vi "circle_measurements.vi"(0 "Radius":dbl) -> (1 "Area":dbl, 2 "Circumference":dbl, 3 "Diameter":dbl)   [LabVIEW 2010]
doc: "Given the radius r, this vi calculates the diameter, circumference, and area of the circle"
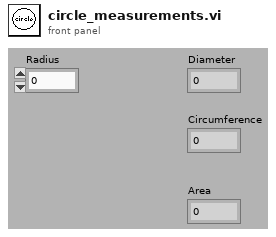
[diagram p1: front panel]
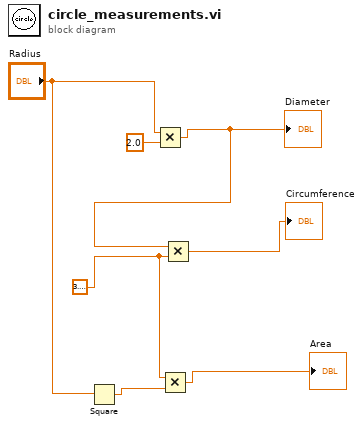
[diagram p0: block diagram]
diagram:
  w3 = 3.141592653589793
  n1 = Square(x="Radius") -> (x^2=w2:dbl)
  n2 = Multiply(x="Radius", y=2.0) -> (x*y=w6:dbl)
  "Diameter" <- w6
  n3 = Multiply(x=w3, y=w2) -> (x*y=→"Area":dbl)
  n4 = Multiply(x=w6, y=w3) -> (x*y=→"Circumference":dbl)
